vi "Search For IMEI.vi"(8 "error in":errorcluster, 9 "IMEI":string, 11 "Array":T1(array[cluster])) -> (0 "error out":errorcluster, 1 "Filenames":string[](array[string]), 3 "Sizes":i32[](array[numeric]))   [LabVIEW 2014]
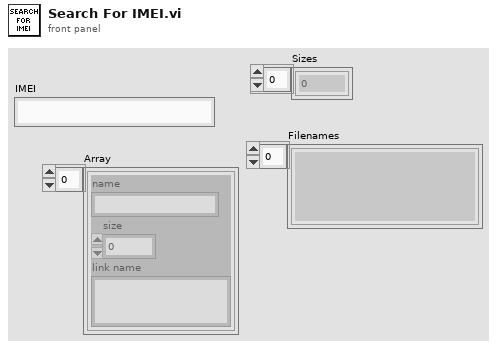
[diagram p1: front panel]
types:
  T1 = cluster{"name":string, "size":i32, "link name":string}[]
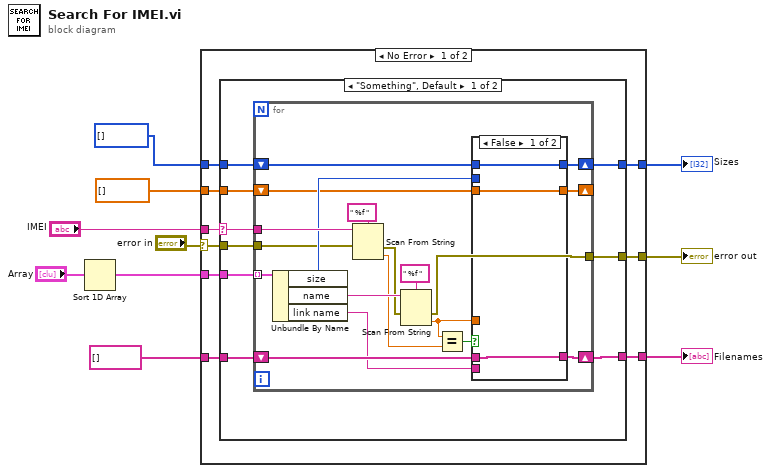
[diagram p0: block diagram]
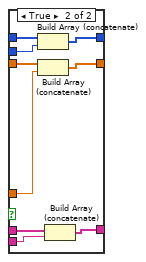
[diagram p2: hidden frame]
diagram:
  n1 = Sort 1D Array(array="Array") -> (sorted array=w8:T1)
  n2 = case shown="No Error" "error in" {
    selector: "error in" -> [w12 w64]
    tunnel: dbl[] [] -> [w19 _]
    tunnel: i32[] [] -> [w18 w63]
    tunnel: w8 -> [w17 _]
    tunnel: [w16 w63] -> w7
    tunnel: string[] [] -> [w15 w62]
    tunnel: [w14 w62] -> w5
    tunnel: "IMEI" -> [w13 _]
    tunnel: [w11 w64] -> w1
    frame No Error {
      n3 = case shown="\"Something\", Default" w13 {
        selector: w13 -> [w22 _]
        tunnel: w19 -> [w28 _]
        tunnel: w18 -> [w27 w60]
        tunnel: w17 -> [w26 _]
        tunnel: [w25 w60] -> w16
        tunnel: w15 -> [w24 w61]
        tunnel: [w23 w61] -> w14
        tunnel: w12 -> [w21 _]
        tunnel: [w20 _] -> w11
        frame "Something", Default {
          n4 = for {
            tunnel: w26 -> [w47] mode=indexing
            tunnel: w22 -> [w43]
            shift-right: [w37] -> w25
            shift-left: w27 -> [w38]
            shift-right: [w35] -> _
            shift-left: w28 -> [w36]
            shift-right: [w32] -> w23
            shift-left: w24 -> [w34]
            tunnel: w21 -> [w30]
            tunnel: [w31] -> w20
            n5 = Unbundle By Name(w47) -> ("size"=w40:i32, "name"=w46:string, "link name"=w33:string)
            n6 = Scan From String(format string=" %f ", input string=w43, error in=w30) -> (error out=w29:errorcluster, output 1=w42:dbl)  [unwired: 2 in, 2 out]
            n7 = Scan From String(format string=" %f ", input string=w46, error in=w29) -> (error out=w31:errorcluster, output 1=w39:dbl)  [unwired: 2 in, 2 out]
            n8 = Equal?(x=w39, y=w42) -> (x = y?=w41:bool)
            n9 = case shown="False" w41 {
              tunnel: w40 -> [_ w58]
              tunnel: w39 -> [_ w59]
              tunnel: w38 -> [w49 w57]
              tunnel: [w49 w56] -> w37
              tunnel: w36 -> [w50 w55]
              tunnel: [w50 w54] -> w35
              tunnel: w34 -> [w48 w52]
              tunnel: w33 -> [_ w51]
              tunnel: [w48 w53] -> w32
              frame False {
              }
              frame True {
                n10 = Build Array (concatenate)(w57, w58) -> (w56:i32[])
                n11 = Build Array (concatenate)(w55, w59) -> (w54:dbl[])
                n12 = Build Array (concatenate)(w52, w51) -> (w53:string[])
              }
            }
          }
        }
        frame "" {
        }
      }
    }
    frame Error {
    }
  }
  "Sizes" <- w7
  "Filenames" <- w5
  "error out" <- w1
